vi "AuMT8852B Power Control Results Query.vi"(8 "error in (no error)":errorcluster, 11 "VISA session":refnum<visa-resource-name>) -> (0 "error out":errorcluster, 2 "error code":i32, 3 "VISA session out":refnum<visa-resource-name>, 4 "Results":T1 {"Average power for each step" format="%.2f"; "Minimum step size" format="%.2f"; "Maximum step size" format="%.2f"; "Minimum power" format="%.2f"; "Maximum power" format="%.2f"; "Current packet average power" format="%.2f"})   [LabVIEW 2017]
doc: "Anritsu MT8852B Bluetooth Tester\n\nReturns the results of the Power Control test.\n\nOUTPUTS\nResults - measurements made during the test."
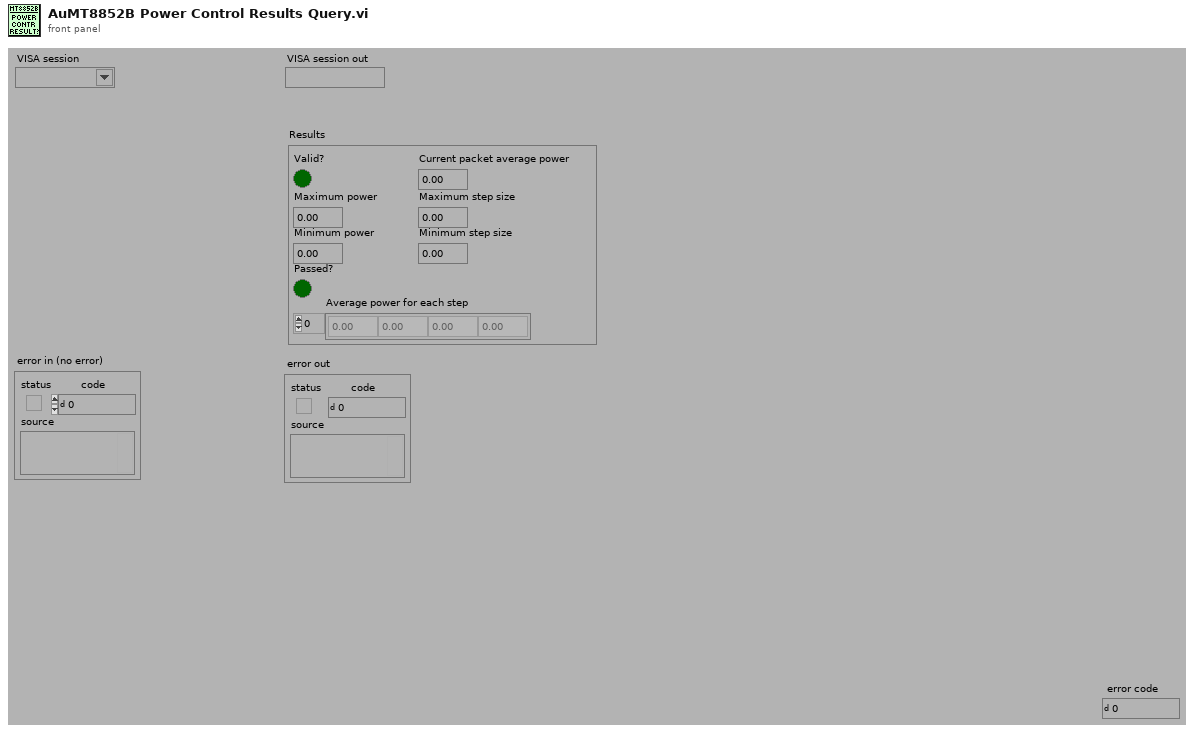
[diagram p1: front panel]
types:
  T1 = cluster{"Current packet average power":dbl, "Maximum power":dbl, "Minimum power":dbl, "Maximum step size":dbl, "Passed?":bool, "Minimum step size":dbl, "Valid?":bool, "Average power for each step":dbl[]}
  T2 = enum16{"Simulate", "Range check", "Cache", "Query instrument status"}
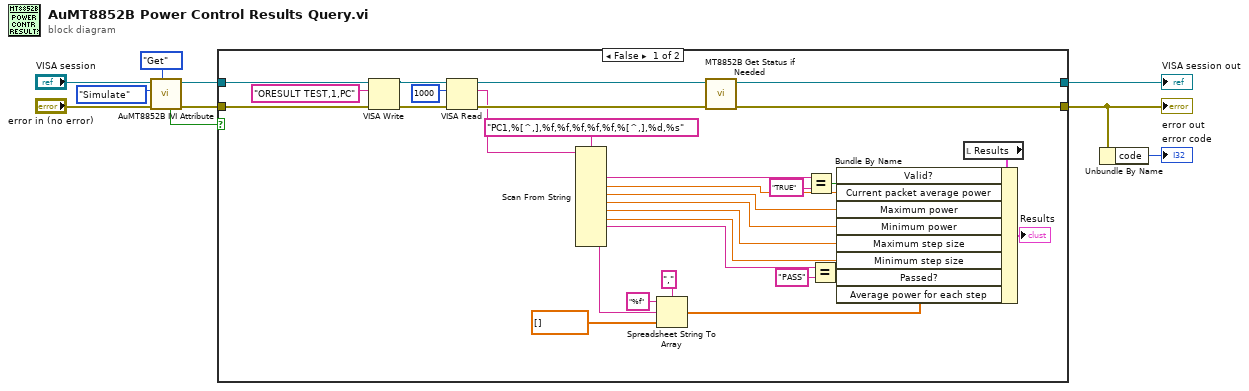
[diagram p0: block diagram]
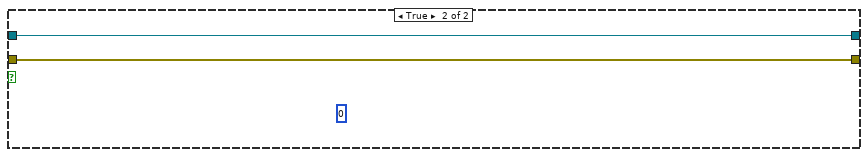
[diagram p2: hidden frame]
diagram:
  n1 = call <instrlib>:"AuMT8852B IVI Attribute.vi"("Set/Get (Set)"=enum16{"Set", "Get"}."Get", "error in (no error)"="error in (no error)", "Flag (Simulate)"=T2."Simulate", "VISA session"="VISA session") -> ("error out"=w7:errorcluster, "VISA session out"=w9:refnum<visa-resource-name>, "Value out"=w3:bool)  [unwired: 5 in]
  n2 = case shown="False" w3 {
    tunnel: [w23 w42] -> w10
    tunnel: [w22 w41] -> w1
    tunnel: w9 -> [w39 w42]
    tunnel: w7 -> [w38 w41]
    frame False {
      n3 = VISA Write(VISA resource name=w39, write buffer="ORESULT TEST,1,PC" ("write buffer (\"\")"), error in (no error)=w38) -> (VISA resource name out=w37:refnum<visa-resource-name>, error out=w36:errorcluster)  [unwired: 1 out]
      n4 = VISA Read(VISA resource name=w37, byte count=u32 1000 ("byte count (0)"), error in (no error)=w36) -> (VISA resource name out=w18:refnum<visa-resource-name>, read buffer=w11:string, error out=w17:errorcluster)  [unwired: 1 out]
      n5 = Scan From String(format string="PC1,%[^,],%f,%f,%f,%f,%f,%[^,],%d,%s" ("Format String"), input string=w11) -> (output 1=w31:string, output 2=w29:dbl, output 3=w28:dbl, output 4=w27:dbl, output 5=w26:dbl, output 6=w19:dbl, output 7=w21:string, output 9=w15:string)  [unwired: 12 in, 3 out]
      n6 = Spreadsheet String To Array(delimiter (Tab)=",", format string="%f", spreadsheet string=w15, array type (2D Dbl)=dbl[] [] ("Array Constant")) -> (array=w12:dbl[])
      n7 = call <instrlib>:"MT8852B Get Status if Needed.vi"("error in (no error)"=w17, "VISA session"=w18) -> ("error out"=w22:errorcluster, "VISA session out"=w23:refnum<visa-resource-name>)  [unwired: 8 in]
      n8 = Equal?(x=w31, y="TRUE") -> (x = y?=w32:bool)
      n9 = Equal?(x=w21, y="PASS") -> (x = y?=w20:bool)
      n10 = local read "Results"() -> (w33:T1)
      n11 = Bundle By Name(cluster=w33, "Valid?"=w32, "Current packet average power"=w29, "Maximum power"=w28, "Minimum power"=w27, "Maximum step size"=w26, "Minimum step size"=w19, "Passed?"=w20, "Average power for each step"=w12) -> (→"Results":T1)
    }
    frame True {
      (unwired) u8 0
    }
  }
  "error out" <- w1
  "VISA session out" <- w10
  n12 = Unbundle By Name(w1) -> ("code"=→"error code":i32)
